vi "A 侧面 处理函数CCD6.vi"(7 "Session Out CCD1":T1, 8 "error in (no error)":errorcluster caption="错误输入（无错误）", 10 "Image Name":string="I1", 11 "CR-字符检测基础参数":T2={"IsNorImage"=TRUE, "Exposure Values"=100289, "ImagePath"=path "C:/Users/hedongpo/Desktop/514-hdp/Alignment Assemble System/Test Picture/B/3.bmp"} caption="参数界面" {"Exposure Values" scale=0.0..200000.0}) -> (0 "error out":errorcluster caption="错误输出", 2 "Session Out":T1, 3 "Image out":T3(plugin-control), 4 "数值":dbl)   [LabVIEW 2017]
uses:
  <vilib>/userdefined/High Color/IMAQdx.ctl
  <vilib>/vision/driver/IMAQdx.llb/IMAQdx Buffer Number Mode.ctl
  Global System.vi
  <vilib>/vision/driver/NI_Vision_Acquisition_Software.lvlib
  <resource>/objmgr/imaqdx.rc
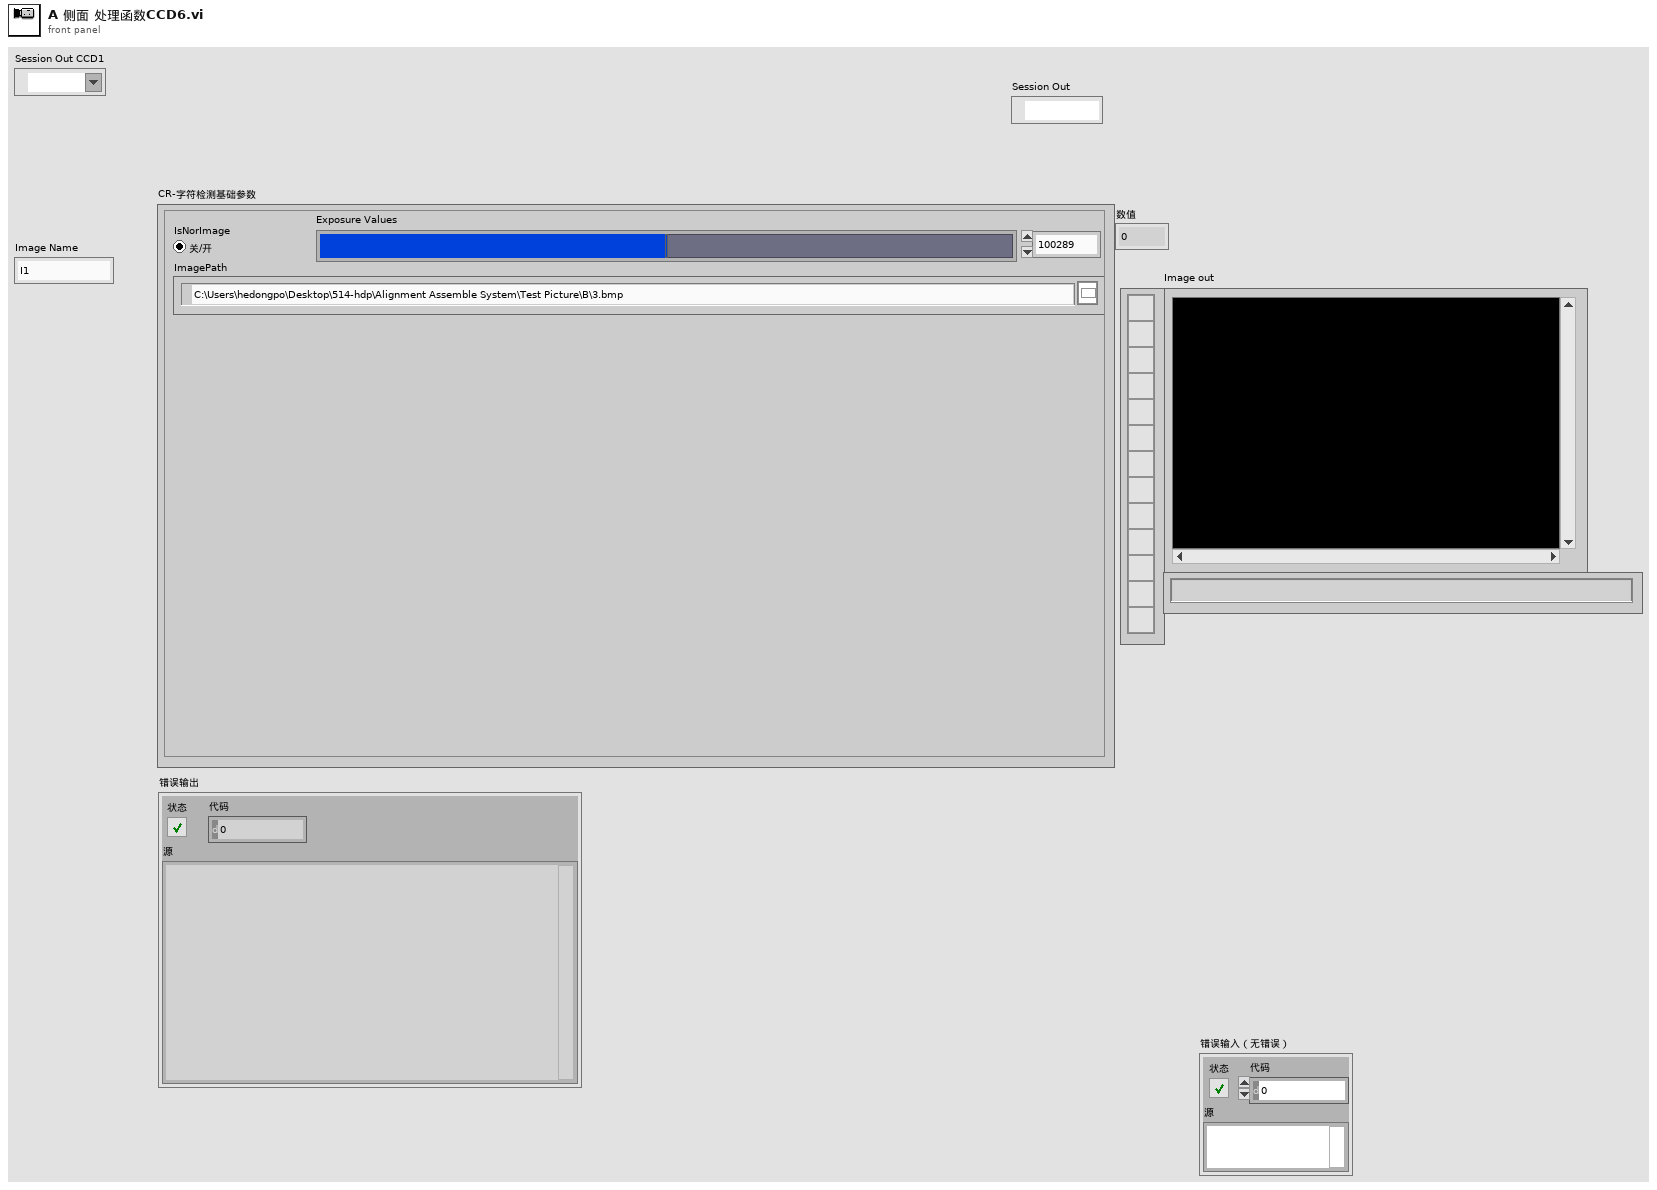
[diagram p1: front panel]
types:
  T1 = typedef "IMAQdx.ctl" = refnum<k21>
  T2 = cluster{"IsNorImage":bool, "Exposure Values":i64, "ImagePath":path}
  T3 = typedef "IMAQ Image.ctl" = refnum<image>
  T4 = typedef "Image Type" = u32
  T5 = typedef "NI_Vision_Acquisition_Software.lvlib/IMAQdx Buffer Number Mode.ctl" = enum32{"Next", "Last", "Buffer Number", "Every", "Last New"}
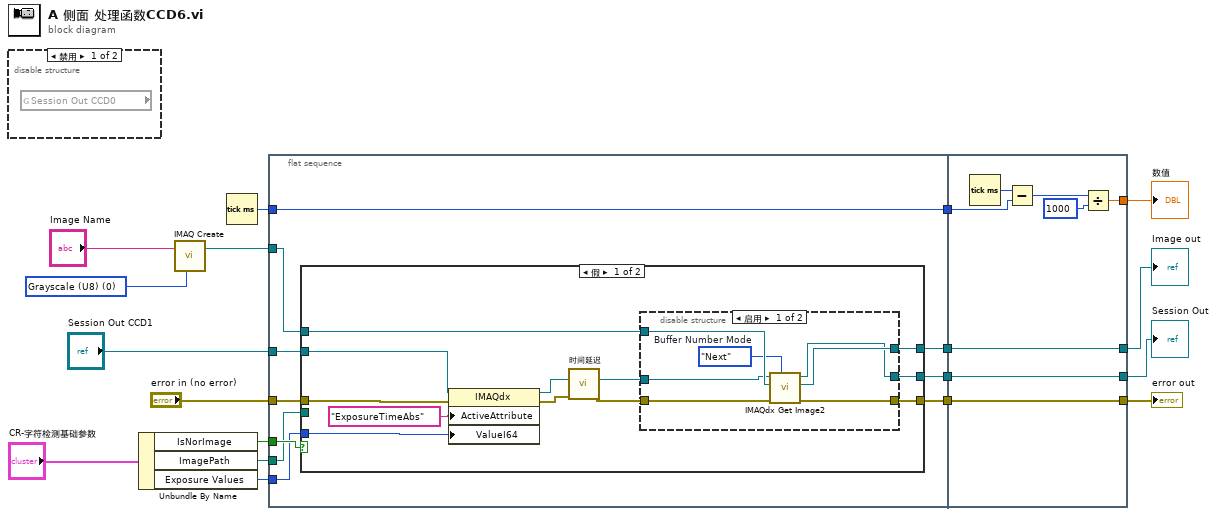
[diagram p0: block diagram]
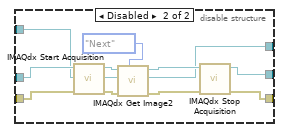
[diagram p3: hidden frame]
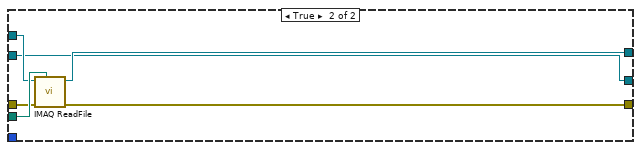
[diagram p4: hidden frame]
diagram:
  w13 = T4 0 items=["Grayscale (U8)", "Grayscale (I16)", "Grayscale (SGL)", "Complex (CSG)", "RGB (U32)", "HSL (U32)", "RGB (U64)", "Grayscale (U16)"] ("Image Type")
  n1 = disable-structure shown="禁用" {
    frame Disabled {
      n2 = global read "Global System.vi" "Session Out CCD0"() -> ()  [unwired: 1 out]
    }
    frame Enabled {
    }
  }
  n3 = Unbundle By Name("CR-字符检测基础参数") -> ("IsNorImage"=w2:bool, "ImagePath"=w3:path, "Exposure Values"=w18:i64)
  n4 = call "IMAQ Create"("Image Name"="Image Name", "Image Type"=w13) -> ("New Image"=w16:T3)  [unwired: 3 in, 1 out]
  n5 = Tick Count (ms)() -> (millisecond timer value=w9:u32)
  n6 = flat-sequence {
    tunnel: w2 -> [w28]
    tunnel: w3 -> [w27]
    tunnel: w18 -> [w26]
    tunnel: w16 -> [w25]
    tunnel: "error in (no error)" -> [w24]
    tunnel: "Session Out CCD1" -> [w21]
    tunnel: w9 -> [w19]
    tunnel: [w23] -> w8
    tunnel: [w22] -> w7
    tunnel: [w20] -> w6
    tunnel: [w19] -> w5
    tunnel: [w69] -> w10
    tunnel: [w70] -> w11
    tunnel: [w71] -> w14
    tunnel: w8 -> [w71]
    tunnel: w7 -> [w70]
    tunnel: w6 -> [w69]
    tunnel: w5 -> [w67]
    tunnel: [w64] -> w4
    frame #0 {
      n7 = case shown="假" w28 {
        tunnel: w27 -> [_ w63]
        tunnel: [w38 w62] -> w22
        tunnel: w26 -> [w32 _]
        tunnel: w21 -> [w34 w58]
        tunnel: w25 -> [w39 w61]
        tunnel: w24 -> [w33 w60]
        tunnel: [w36 w59] -> w23
        tunnel: [w37 w58] -> w20
        frame False {
          n8 = property class="IMAQdx"(reference=w34, error in=w33, "ActiveAttribute"="ExposureTimeAbs", "ValueI64"=w32) -> (reference out=w35:T1, error out=w31:errorcluster)
          n9 = call "时间延迟"("error in (no error)"=w31) -> ("error out"=w29:errorcluster)  [unwired: 10 in]
          n10 = disable-structure shown="启用" {
            disable-tunnel: w39 -> [w46 w50]
            disable-tunnel: [w45 w48] -> w38
            disable-tunnel: [w44 w47] -> w37
            disable-tunnel: [w43 w49] -> w36
            disable-tunnel: w35 -> [w42 w51]
            disable-tunnel: w29 -> [w40 w52]
            frame Enabled {
              w41 = IMAQdx_Buffer_Number_Mode."Next"  # Buffer Number Mode
              n11 = call <vilib>:"IMAQdx Get Image2.vi"("Buffer Number Mode (Next)"=w41, "error in"=w40, "Image In"=w46, "Session In"=w42) -> ("error out"=w43:errorcluster, "Image Out"=w45:T3, "Session Out"=w44:T1)  [unwired: 4 in, 1 out]
            }
            frame Disabled {
              n12 = call <vilib>:"IMAQdx Start Acquisition.vi"("error in"=w52, "Session In"=w51) -> ("error out"=w54:errorcluster, "Session Out"=w55:T1)  [unwired: 8 out]
              n13 = call <vilib>:"IMAQdx Get Image2.vi"("Buffer Number Mode (Next)"=IMAQdx_Buffer_Number_Mode."Next" ("Buffer Number Mode"), "error in"=w54, "Image In"=w50, "Session In"=w55) -> ("error out"=w56:errorcluster, "Image Out"=w48:T3, "Session Out"=w57:T1)  [unwired: 4 in, 1 out]
              n14 = call <vilib>:"IMAQdx Stop Acquisition.vi"("error in"=w56, "Session In"=w57) -> ("error out"=w49:errorcluster, "Session Out"=w47:T1)  [unwired: 8 out]
            }
          }
        }
        frame True {
          n15 = call "IMAQ ReadFile"("File Path"=w63, "error in (no error)"=w60, "Image"=w61) -> ("error out"=w59:errorcluster, "Image Out"=w62:T3)  [unwired: 4 in, 3 out]
        }
      }
    }
    frame #1 {
      n16 = Tick Count (ms)() -> (millisecond timer value=w68:u32)
      n17 = Subtract(x=w68, y=w67) -> (x-y=w66:u32)
      n18 = Divide(x=w66, y=u32 1000) -> (x/y=w64:dbl)
    }
  }
  "Image out" <- w11
  "error out" <- w14
  "Session Out" <- w10
  "数值" <- w4
